vi "ryTimerEx Queue Performance.vi"() -> ()   [LabVIEW 2020]
uses:
  3122cb75-6530-49f8-9864-937ee694b227.vi
panel:
  out "Chart":cluster{dbl, i32}(graph)
  out "Delta Ticks (ms)":i32
  out "Counter":u32
  out "Error":errorcluster
  out "Delta (ms)":dbl format="%.4f"
  in  "Exit":bool
  # "Repeats the \"MSG1\"\nevery second."
  # "Plots the delta time (Tick counts &\nhigh precision) to see the OS jitter."
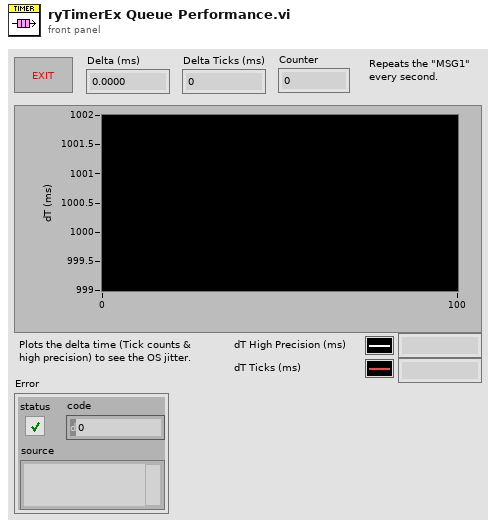
[diagram p1: front panel]
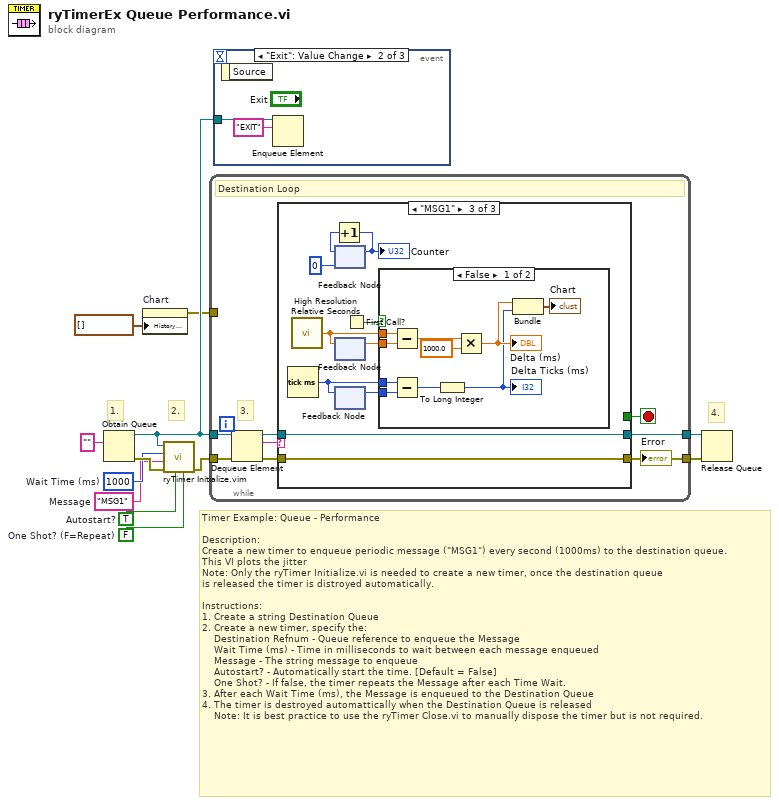
[diagram p0: block diagram]
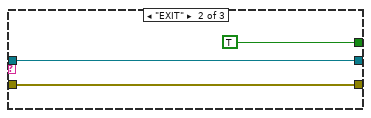
[diagram p3: hidden frame]
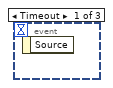
[diagram p5: hidden frame]
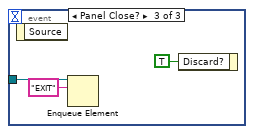
[diagram p6: hidden frame]
diagram:
  w1 = FALSE  # One Shot? (F=Repeat)
  w8 = TRUE  # Autostart?
  w9 = "MSG1"  # Message
  w10 = u32 1000  # Wait Time (ms)
  # "Timer Example: Queue - Performance\n\nDescription:\nCreate a new timer to enqueue periodic message (\"MSG1\") every second (1000ms) to the destination queue.\nThis VI plots the jitter\nNote: Only the ryTimer Initialize.vi is needed to create a new timer, once the destination queue\nis released the timer is distroyed automatically.\n\nInstructions:\n1. Create a string Destination Queue\n2. Create a new timer, specify the:\n    Destination Refnum - Queue reference to enqueue the Message\n    Wait Time (ms) - Time in milliseconds to wait between each message enqueued\n    Message - The string message to enqueue\n    Autostart? - Automatically start the time. [Default = False]\n    One Shot? - If false, the timer repeats the Message after each Time Wait.\n3. After each Wait Time (ms), the Message is enqueued to the Destination Queue\n4. The timer is destroyed automattically when the Destination Queue is released\n    Note: It is best practice to use the ryTimer Close.vi to manually dispose the timer but is not required."
  # "4."
  # "2."
  # "1."
  n1 = Obtain Queue(element data type="") -> (queue out=w4:refnum<queue>, error out=w11:errorcluster)  [unwired: 4 in, 1 out]
  n2 = property on="Chart" class="WFChart (strict)"("History Data"=cluster{dbl, i32}[] []) -> (error out=w3:errorcluster)  [unwired: 2 in, 1 out]
  n3 = call "ryTimer Initialize.vim"("One Shot? (F=Repeat)"=w1, "Autostart? (F)"=w8, "error in (no error)"=w11, "Message"=w9, "Wait Time (ms)"=w10, "Destination Refnum [Q,UE,Any]"=w4) -> ("error out"=w6:errorcluster)  [unwired: 4 in, 1 out]
  n4 = while {
    tunnel: w4 -> [w20]
    tunnel: [w18] -> w7
    tunnel: w6 -> [w16]
    tunnel: [w13] -> w5
    tunnel: w3 -> [_]
    stop <- w14 stop-if-true
    # "3."
    # "Destination Loop"
    n5 = Dequeue Element(queue=w20, error in (no error)=w16) -> (queue out=w17:refnum<queue>, element=w19:string, error out=w15:errorcluster)  [unwired: 1 in, 1 out]
    n6 = case shown="\"MSG1\"" w19 {
      tunnel: [w22 w25 w35] -> w18
      tunnel: w17 -> [w22 w25 w35]
      tunnel: [w21 w24 w34] -> w13
      tunnel: w15 -> [w21 w24 w34]
      tunnel: [_ TRUE _] -> w14
      frame Default {
      }
      frame "EXIT" {
      }
      frame "MSG1" {
        n7 = Tick Count (ms)() -> (millisecond timer value=w28:u32)
        n8 = call <vilib>:"High Resolution Relative Seconds.vi"() -> ("relative seconds"=w32:dbl)
        n9 = feedback #1(u32 0 ("millisecond timer value")) -> (w30:u32)
        n10 = Increment(x=w30) -> (x+1=w29:u32)
        "Counter" <- w29
        n11 = feedback-in #1(w29) -> ()
        n12 = feedback-in #2(w32) -> ()
        n13 = feedback #2() -> (w33:dbl)  [unwired: 1 in]
        n14 = feedback #3() -> (w27:u32)  [unwired: 1 in]
        n15 = feedback-in #3(w28) -> ()
        n16 = First Call?() -> (First Call?: T/F=w26:bool)
        n17 = case shown="False" w26 {
          tunnel: w33 -> [w45 _]
          tunnel: w32 -> [w44 _]
          tunnel: w28 -> [w43 _]
          tunnel: w27 -> [w42 _]
          frame False {
            n18 = Subtract(x=w44, y=w45) -> (x-y=w38:dbl)
            n19 = Subtract(x=w43, y=w42) -> (x-y=w36:u32)
            n20 = To Long Integer(number=w36) -> (32bit integer=w39:i32)
            "Delta Ticks (ms)" <- w39
            n21 = Multiply(x=w38, y=1000.0) -> (x*y=w41:dbl)
            "Delta (ms)" <- w41
            n22 = Bundle(w41, w39) -> (→"Chart":cluster{dbl, i32})  [unwired: 1 in]
          }
          frame True {
          }
        }
      }
    }
    "Error" <- w13
  }
  n23 = event shown="[1] \"Exit\": Value Change" {
    selector: _ -> [_ _ _]
    dyn-events: _ -> [_ _ _]
    timeout: _ -> [_ _ _]
    tunnel: w4 -> [_ w47 w50]
    event Timeout {
      n24 = event-data() -> ()  [unwired: 1 in, 1 out]
    }
    event "Exit": Value Change {
      n25 = event-data() -> ()  [unwired: 1 in, 1 out]
      n26 = Enqueue Element(queue=w47, element="EXIT") -> ()  [unwired: 2 in, 3 out]
    }
    event Panel Close? {
      n27 = event-data() -> ()  [unwired: 1 in, 1 out]
      n28 = Enqueue Element(queue=w50, element="EXIT") -> ()  [unwired: 2 in, 3 out]
      n29 = event-data("Discard?"=TRUE) -> ()  [unwired: 1 in, 1 out]
    }
  }
  n30 = Release Queue(queue=w7, error in (no error)=w5) -> ()  [unwired: 1 in, 3 out]
